vi "BRig_RT_storeData__1D_u16.vi"(10 "Array":u16[](array[numeric]), 11 "input_filename":string) -> ()   [LabVIEW 2014]
uses:
  <vilib>/Utility/file.llb/Write To Spreadsheet File (DBL).vi
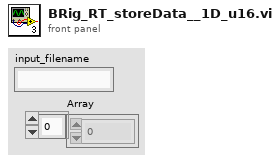
[diagram p1: front panel]
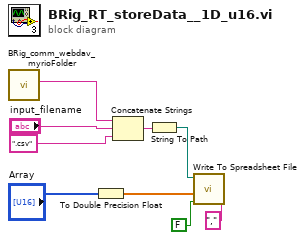
[diagram p0: block diagram]
diagram:
  n1 = call "BRig_comm_webdav_myrioFolder.vi"() -> ("output_myrioFolder"=w6:string)  [unwired: 11 in]
  n2 = To Double Precision Float(number="Array") -> (double precision float=w1:dbl[])
  n3 = Concatenate Strings(w6, "input_filename", ".csv" ("string")) -> (w4:string)
  n4 = String To Path(string=w4) -> (path=w3:path)
  n5 = call-poly <vilib>:"Write To Spreadsheet File.vi"("delimiter (\\t)"="," ("delimiter (\\t)"), "append to file? (new file:F)"=FALSE, "1D data"=w1, "file path (dialog if empty)"=w3) -> ()  [unwired: 4 in, 1 out]
